vi "Wheel Speed Selection.vi"(9 "D4?":bool, 10 "Numeric Control":u32, 11 "Shooter Data":T1) -> (1 "Flashlight":bool, 2 "Intake Speed":dbl, 3 "Shooter Speed":dbl)   [LabVIEW 2015]
uses:
  <vilib>/Rock Robotics/Network Tables/NT Read Number.vi
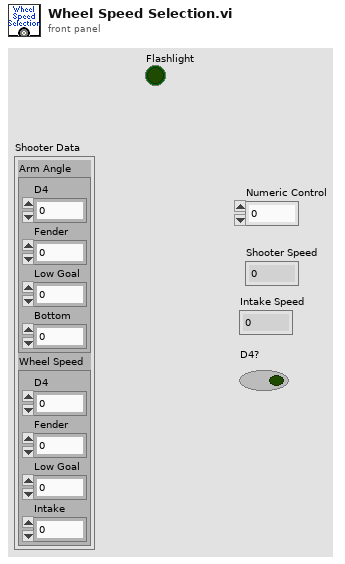
[diagram p1: front panel]
types:
  T1 = cluster{"Arm Angle":cluster{"D4":dbl, "Fender":dbl, "Low Goal":dbl, "Bottom":dbl}, "Wheel Speed":cluster{"D4":dbl, "Fender":dbl, "Low Goal":dbl, "Intake":dbl}}
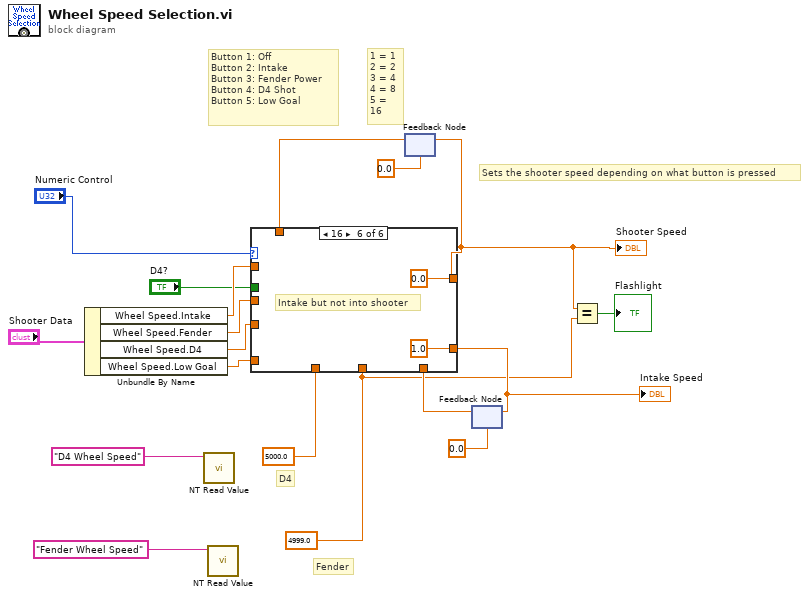
[diagram p0: block diagram]
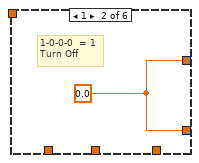
[diagram p3: hidden frame]
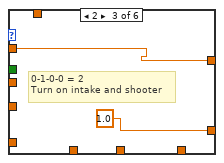
[diagram p4: hidden frame]
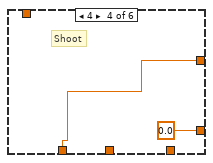
[diagram p5: hidden frame]
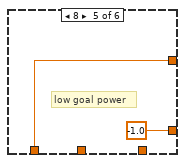
[diagram p6: hidden frame]
diagram:
  w1 = 4999.0 ("Numeric")
  # "D4"
  # "Fender"
  # "1 = 1\n2 = 2\n3 = 4\n4 = 8\n5 = 16"
  # "Sets the shooter speed depending on what button is pressed"
  # "Button 1: Off\nButton 2: Intake \nButton 3: Fender Power \nButton 4: D4 Shot\nButton 5: Low Goal"
  n1 = Unbundle By Name("Shooter Data") -> ("Wheel Speed.Intake"=w11:dbl, "Wheel Speed.Fender"=w10:dbl, "Wheel Speed.D4"=w9:dbl, "Wheel Speed.Low Goal"=w8:dbl)
  n2 = call-poly <vilib>:"NT Read Value.vi"("Name"="D4 Wheel Speed") -> ()  [unwired: 9 in, 2 out]
  n3 = call-poly <vilib>:"NT Read Value.vi"("Name"="Fender Wheel Speed") -> ()  [unwired: 9 in, 2 out]
  n4 = feedback #1(0.0) -> (w14:dbl)
  n5 = feedback #2(0.0) -> (w15:dbl)
  n6 = case shown="16" "Numeric Control" {
    tunnel: [w19 w21 w22 w24 w26 0.0 ("Low Goal")] -> w4
    tunnel: [w20 w21 1.0 0.0 -1.0 1.0] -> w12
    tunnel: w15 -> [w20 _ _ _ _ _]
    tunnel: w14 -> [w19 _ _ _ _ _]
    tunnel: w11 -> [_ _ w22 _ _ _]
    tunnel: w10 -> [_ _ _ _ _ _]
    tunnel: w9 -> [_ _ _ _ _ _]
    tunnel: w8 -> [_ _ _ _ _ _]
    tunnel: 5000.0 -> [_ _ _ w24 w26 _]
    tunnel: w1 -> [_ _ _ _ _ _]
    tunnel: "D4?" -> [_ _ _ _ _ _]
    frame 0, Default {
      # "0-0-0-0 = 0\nStay at current speed"
    }
    frame 1 {
      w21 = 0.0
      # "1-0-0-0  = 1\nTurn Off"
    }
    frame 2 {
      # "0-1-0-0 = 2\nTurn on intake and shooter"
    }
    frame 4 {
      # "Shoot"
    }
    frame 8 {
      # "low goal power"
    }
    frame 16 {
      # "Intake but not into shooter"
    }
  }
  "Shooter Speed" <- w4
  "Intake Speed" <- w12
  n7 = feedback-in #1(w4) -> ()
  n8 = feedback-in #2(w12) -> ()
  n9 = Equal?(x=w4, y=w1) -> (x = y?=→"Flashlight":bool)
